vi "Set Values.vi"(8 "error in (no error)":errorcluster, 10 "Delay Time":dbl, 11 "Time Step in":refnum<class "Time Step.lvclass">) -> (0 "error out":errorcluster, 3 "Time Step out":refnum<class "Time Step.lvclass">)   [LabVIEW 2018, in "Temp Recipe.lvlib" / "Time Step.lvclass"]
uses:
  Time Step.lvclass
  C:/dev/source/Systems/NI Week/Temperature Recipe/Temp Recipe/Recipe Step/Recipe Step.lvclass
  Time Step.lvclass/Time Step.ctl
  Recipe Step/Recipe Step.lvclass
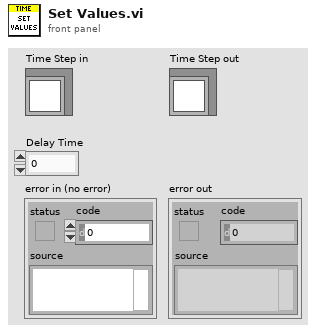
[diagram p1: front panel]
types:
  T1 = typedef "Temp Recipe.lvlib/Time Step.lvclass/Ref Data.ctl" = cluster{"Delay Time (S)":dbl}
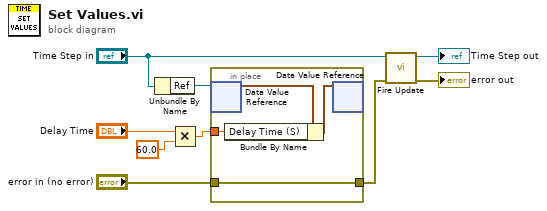
[diagram p0: block diagram]
diagram:
  n1 = Unbundle By Name("Time Step in") -> ("Ref"=w9:refnum<data-value>)
  n2 = Multiply(x="Delay Time", y=60.0) -> (x*y=w2:dbl)
  n3 = in-place {
    in-place-border: w2 -> [w11]
    in-place-border: "error in (no error)" -> [w10]
    in-place-border: [w10] -> w8
    n4 = in-place-dvr #1(w9) -> (w13:T1)  [unwired: 1 out]
    n5 = Bundle By Name(cluster=w13, "Delay Time (S)"=w11) -> (w12:T1)
    n6 = in-place-dvr #1(w12) -> ()  [unwired: 2 out]
  }
  n7 = call "Fire Update.vi"("error in (no error)"=w8, "Recipe Step in"="Time Step in") -> ("error out"=→"error out":errorcluster, "Recipe Step out"=→"Time Step out":refnum<class "Time Step.lvclass">)  [unwired: 8 in]
